vi "SV Open Work Sheet.vi"(2 "error in (no error)":errorcluster, 3 "Sheet":variant, 4 "Refnum Cluster In":T1) -> (0 "error out":errorcluster, 1 "Refnum Cluster Out":T2)   [LabVIEW 2010]
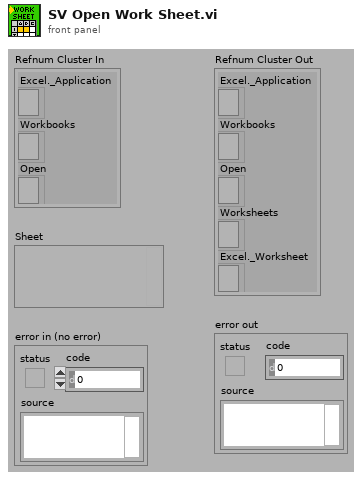
[diagram p1: front panel]
types:
  T1 = cluster{"Excel._Application":refnum<k7>, "Workbooks":refnum<k7>, "Open":refnum<k7>}
  T2 = cluster{"Excel._Application":refnum<k7>, "Workbooks":refnum<k7>, "Open":refnum<k7>, "Worksheets":refnum<k7>, "Excel._Worksheet":refnum<k7>}
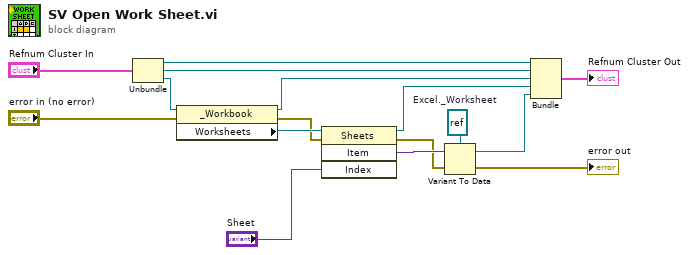
[diagram p0: block diagram]
diagram:
  w7 = refnum<k7> refnum  # Excel._Worksheet
  n1 = Unbundle("Refnum Cluster In") -> ("Excel._Application"=w12:refnum<k7>, "Workbooks"=w11:refnum<k7>, "Open"=w13:refnum<k7>)
  n2 = property class="_Workbook"(reference=w13, error in="error in (no error)") -> (reference out=w3:refnum<k7>, error out=w6:errorcluster, "Worksheets"=w9:refnum<k7>)
  n3 = invoke class="Sheets" method="Item"(reference=w9, error in=w6, "Index"="Sheet") -> (reference out=w2:refnum<k7>, error out=w5:errorcluster, "Item"=w8:variant)  [unwired: 1 in, 1 out]
  n4 = Variant To Data(error in=w5, Variant=w8, type=w7) -> (error out=→"error out":errorcluster, data=w1:refnum<k7>)
  n5 = Bundle("Excel._Application"=w12, "Workbooks"=w11, "Open"=w3, "Worksheets"=w2, "Excel._Worksheet"=w1) -> (→"Refnum Cluster Out":T2)  [unwired: 1 in]
